vi "Rotate WayPt for Extra Arc.vi"(6 "Pt 0":cluster{"x":dbl, "y":dbl, "th":dbl}, 8 "Blends In":T1[](array[typedef]), 10 "Pts":cluster{"x":dbl, "y":dbl, "th":dbl}[](array[cluster]), 11 "index":i32) -> (0 "Blends Out":T1[](array[typedef]), 1 "Pt2 vertex dist":dbl, 2 "Pt0 vertex dist":dbl, 3 "Pt Out":cluster{"x":dbl, "y":dbl, "th":dbl})   [LabVIEW 2018]
uses:
  BlendType.ctl
panel:
  out "XY Graph":cluster{"X":dbl, "Y":dbl}[](graph)
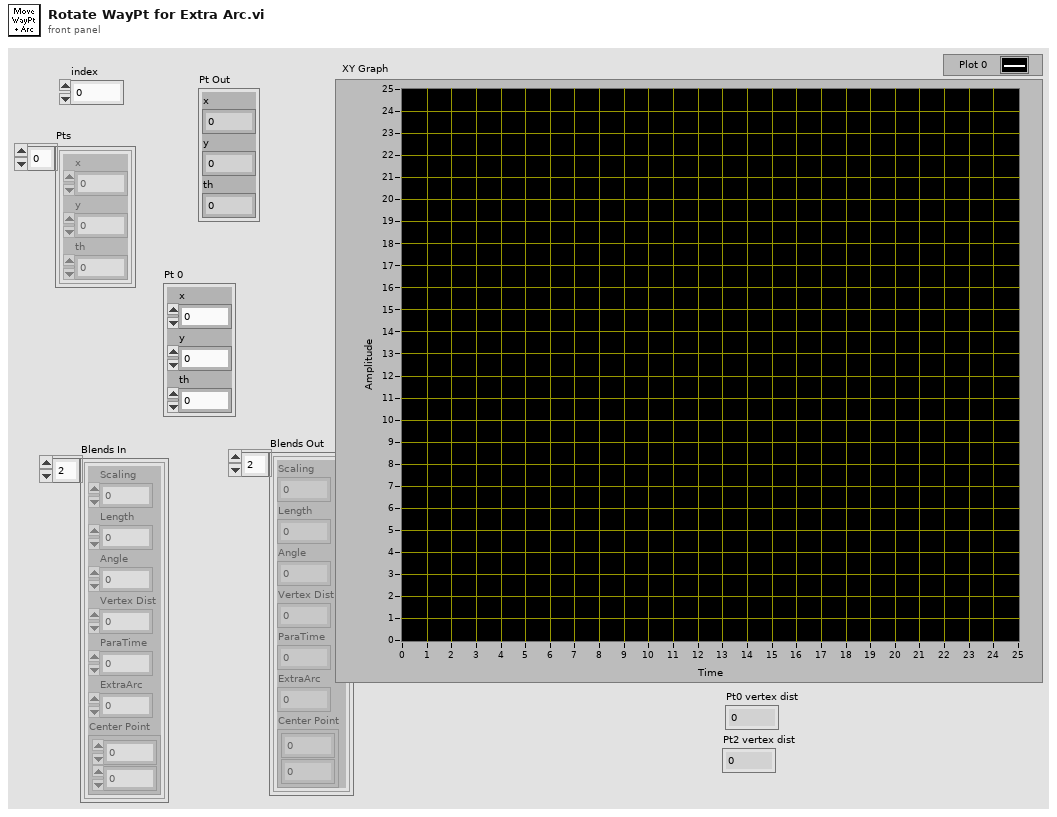
[diagram p1: front panel]
types:
  T1 = typedef "BlendType.ctl" = cluster{"Scaling":dbl, "Length":dbl, "Angle":dbl, "Vertex Dist":dbl, "ParaTime":dbl, "ExtraArc":dbl, "Center Point":cluster{dbl, dbl}}
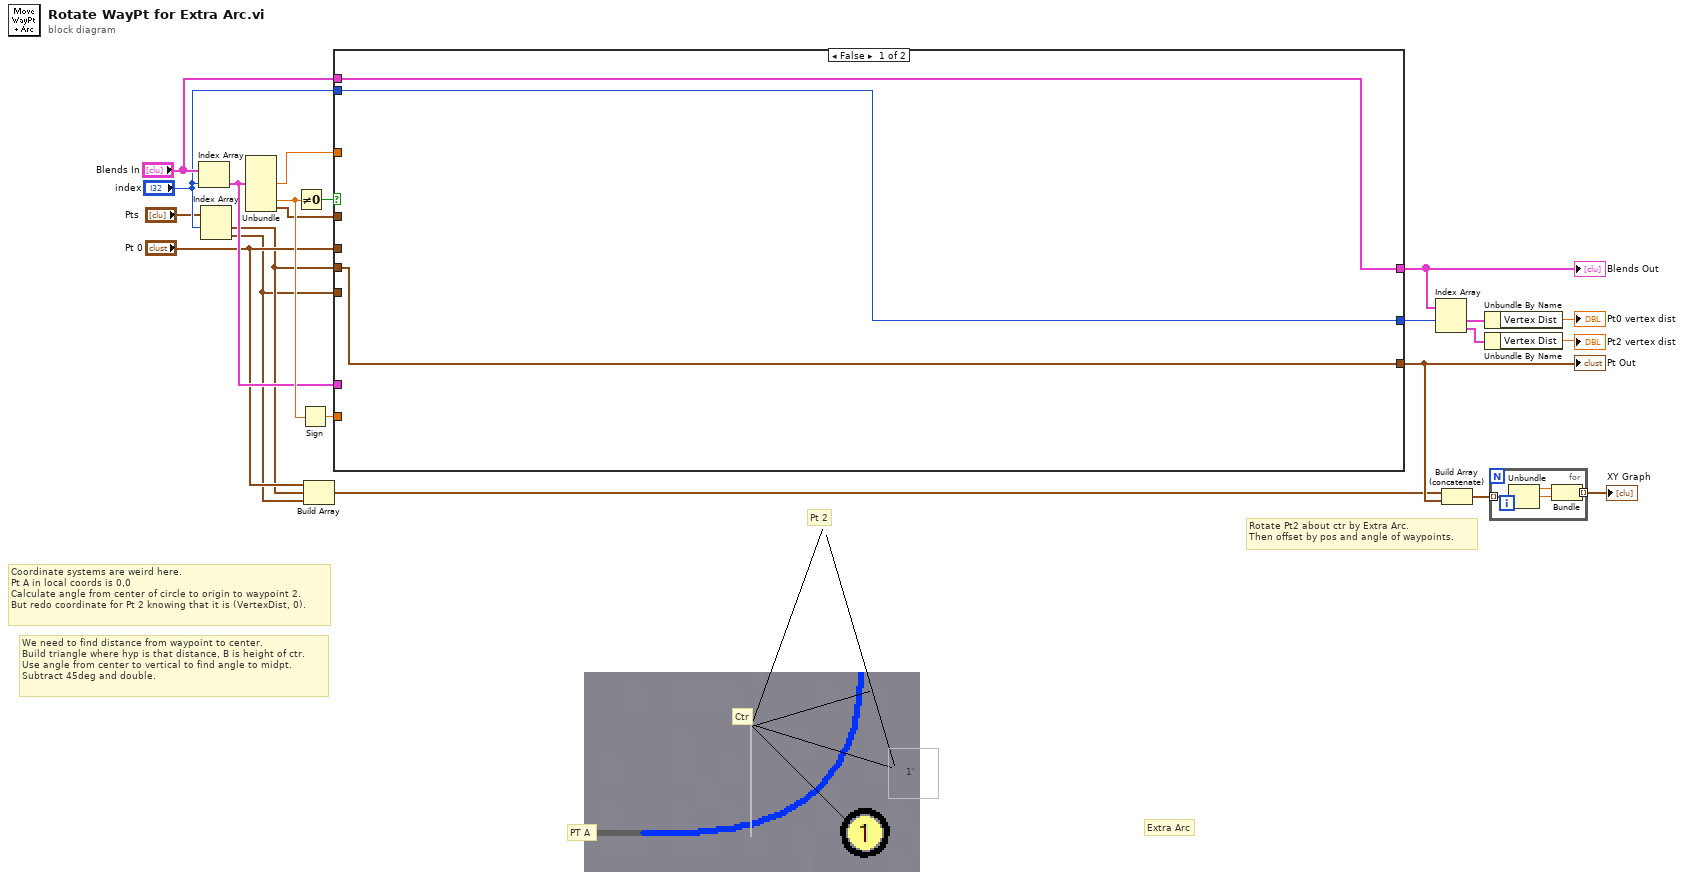
[diagram p0: block diagram]
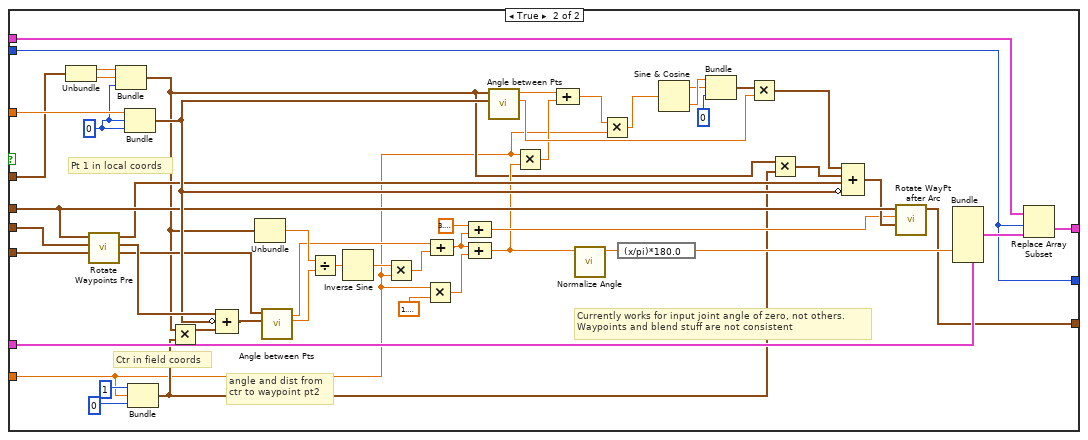
[diagram p2: hidden frame]
diagram:
  # "1'"
  # "We need to find distance from waypoint to center.\nBuild triangle where hyp is that distance, B is height of ctr.\nUse angle from center to vertical to find angle to midpt.\nSubtract 45deg and double."
  # "Extra Arc"
  # "Rotate Pt2 about ctr by Extra Arc.\nThen offset by pos and angle of waypoints."
  # "Ctr"
  # "Pt 2"
  # "PT A"
  # "Coordinate systems are weird here.\nPt A in local coords is 0,0\nCalculate angle from center of circle to origin to waypoint 2.\nBut redo coordinate for Pt 2 knowing that it is (VertexDist, 0)."
  n1 = Index Array(array="Blends In", index="index") -> (element=w14:T1)
  n2 = Index Array(array="Pts", index #1="index") -> (element #1=w4:cluster{"x":dbl, "y":dbl, "th":dbl}, element #2=w3:cluster{"x":dbl, "y":dbl, "th":dbl})  [unwired: 1 in]
  n3 = Unbundle(w14) -> ("Vertex Dist"=w21:dbl, "ExtraArc"=w20:dbl, "Center Point"=w15:cluster{dbl, dbl})  [unwired: 4 out]
  n4 = Not Equal To 0?(x=w20) -> (x != 0?=w22:bool)
  n5 = Sign(1:w20) -> (0:w19:dbl)
  n6 = Build Array("Pt 0", w4, w3) -> (w2:cluster{"x":dbl, "y":dbl, "th":dbl}[])
  n7 = case shown="False" w22 {
    tunnel: w3 -> [_ w27]
    tunnel: [w25 w28] -> w16
    tunnel: w4 -> [w25 w47]
    tunnel: w14 -> [_ w69]
    tunnel: [w24 w26] -> w8
    tunnel: w21 -> [_ w62]
    tunnel: "Pt 0" -> [_ w54]
    tunnel: w19 -> [_ w33]
    tunnel: w15 -> [_ w32]
    tunnel: "Blends In" -> [w24 w31]
    tunnel: "index" -> [w23 w29]
    tunnel: [w23 w29] -> w7
    frame False {
    }
    frame True {
      w61 = 0
      # "angle and dist from\nctr to waypoint pt2"
      # "Pt 1 in local coords"
      # "Currently works for input joint angle of zero, not others.\nWaypoints and blend stuff are not consistent"
      # "Ctr in field coords"
      n8 = Unbundle(w32) -> (w64:dbl, w63:dbl)
      n9 = call "Rotate Waypoints Pre.vi"("Pt 2"=w27, "Pt 1"=w47, "Pt 0"=w54) -> ("Pt 2 out"=w57:cluster{dbl, dbl, dbl}, "Pt 1 out"=w60:cluster{"Vertex Dist":dbl, dbl, dbl}, "Pt 1 rel to Pt0"=w52:cluster{"Vertex Dist":dbl, dbl, dbl})  [unwired: 6 in]
      n10 = Bundle(w64, w63, w61) -> (w38:cluster{dbl, dbl, i32})  [unwired: 1 in]
      n11 = Bundle("Vertex Dist"=w62, w61, w61) -> (w59:cluster{"Vertex Dist":dbl, i32, i32})  [unwired: 1 in]
      n12 = Bundle(1, w33, 0) -> (w34:cluster{i32, dbl, i32})  [unwired: 1 in]
      n13 = Multiply(x=w38, y=w34) -> (x*y=w37:cluster{dbl, dbl, i32})
      n14 = Compound Arithmetic op=ADD(w60, invert w59, w37) -> (w58:cluster{dbl, dbl, dbl})
      n15 = Unbundle(w38) -> (w70:dbl)  [unwired: 2 out]
      n16 = call "Angle between Pts.vi"("Pt 2"=w58, "Pt 1"=w57) -> ("Distance ft"=w56:dbl, "Angle rad"=w55:dbl)  [unwired: 8 in]
      n17 = Divide(x=w70, y=w56) -> (x/y=w49:dbl)
      n18 = Inverse Sine(1:w49) -> (0:w44:dbl)
      n19 = Multiply(x=w44, y=w33) -> (x*y=w43:dbl)
      n20 = Multiply(x=w33, y=1.5707963267948966) -> (x*y=w51:dbl)
      n21 = Compound Arithmetic op=ADD(w55, w43) -> (w66:dbl)
      n22 = Compound Arithmetic op=ADD(3.141592653589793, w66) -> (w48:dbl)
      n23 = Compound Arithmetic op=ADD(w66, w51) -> (w45:dbl)
      n24 = call "Angle between Pts.vi"("Pt 2"=w59, "Pt 1"=w38) -> ("Distance ft"=w71:dbl, "Angle rad"=w76:dbl)  [unwired: 8 in]
      n25 = Multiply(x=w33, y=w45) -> (x*y=w46:dbl)
      n26 = Compound Arithmetic op=ADD(w76, w46) -> (w42:dbl)
      n27 = call "Normalize Angle.vi"("Angle in r"=w45) -> ("Angle out r"=w65:dbl)  [unwired: 10 in]
      n28 = Multiply(x=w42, y=w33) -> (x*y=w41:dbl)
      n29 = expression code="(x/pi)*180.0" ("radians to degrees")(w65) -> (w68:dbl)
      n30 = Sine & Cosine(0:w41) -> (1:w73:dbl, 2:w74:dbl)
      n31 = Bundle(w74, w73, 0) -> (w72:cluster{dbl, dbl, i32})  [unwired: 1 in]
      n32 = Multiply(x=w72, y=w71) -> (x*y=w39:cluster{dbl, dbl, dbl})
      n33 = Multiply(x=w38, y=w34) -> (x*y=w40:cluster{dbl, dbl, i32})
      n34 = Compound Arithmetic op=ADD(w39, w40, w52, invert w59) -> (w53:cluster{dbl, dbl, dbl})
      n35 = call "Rotate WayPt after Arc.vi"("Phantom Waypoint"=w53, "Waypoint Line rad"=w48, "Pt 0"=w54) -> ("Phantom Waypoint out"=w28:cluster{"x":dbl, "y":dbl, "th":dbl})  [unwired: 8 in]
      n36 = Bundle(cluster=w69, "ExtraArc"=w68) -> (w30:T1)  [unwired: 6 in]
      n37 = Replace Array Subset(array=w31, new element=w30, index=w29) -> (w26:T1[])
    }
  }
  "Pt Out" <- w16
  "Blends Out" <- w8
  n38 = Index Array(array=w8, index #1=w7) -> (element #1=w12:T1, element #2=w11:T1)  [unwired: 1 in]
  n39 = Build Array (concatenate)(w2, w16) -> (w18:cluster{"x":dbl, "y":dbl, "th":dbl}[])
  n40 = Unbundle By Name(w12) -> ("Vertex Dist"=→"Pt0 vertex dist":dbl)
  n41 = Unbundle By Name(w11) -> ("Vertex Dist"=→"Pt2 vertex dist":dbl)
  n42 = for {
    tunnel: w18 -> [w78] mode=indexing
    tunnel: [w77] -> w17 mode=indexing
    n43 = Unbundle(w78) -> ("x"=w80:dbl, "y"=w79:dbl)  [unwired: 1 out]
    n44 = Bundle("x"=w80, "y"=w79) -> (w77:cluster{"x":dbl, "y":dbl})  [unwired: 1 in]
  }
  "XY Graph" <- w17
